vi "test_bench.vi"   [LabVIEW 2016]
types:
  T1 = cluster{"B":dbl[][], "Cline":dbl[][], "Kline":dbl[][], "Mline":dbl[][], "Alp0":dbl, "Alp1":dbl, "Gam0":dbl, "Gam1":dbl, "T_shift":dbl, "Numerator":dbl[], "Denominator":dbl[]}
  T2 = typedef "NI_LinSys_Model Typedefs.lvlib/CD State Space Model (MIMO).ctl" = cluster{"properties":T3, "A":dbl[][], "B":dbl[][], "C":dbl[][], "D":dbl[][], "StateNames":string[], "Transport Delay":dbl[][]}
  T3 = typedef "NI_LinSys_Model Typedefs.lvlib/CD General Elements.ctl" = cluster{"Model name":string, "Input names":string[], "Output names":string[], "Input Delays":dbl[], "Output Delays":dbl[], "Sampling Time":dbl, "Notes":string}
  T4 = typedef "NI_LinSys_Model Typedefs.lvlib/CD Transfer Function Model (MIMO).ctl" = cluster{"properties":T3, "transfer function(s)":T5[][]}
  T5 = typedef "NI_LinSys_Model Typedefs.lvlib/CD Transfer Function Model (SISO).ctl" = cluster{"Numerator":dbl[], "Denominator":dbl[], "delay":dbl}
  T6 = cluster{"SysD":T2, "sysDo":T2, "sysDi":T2, "sysDC":T4}
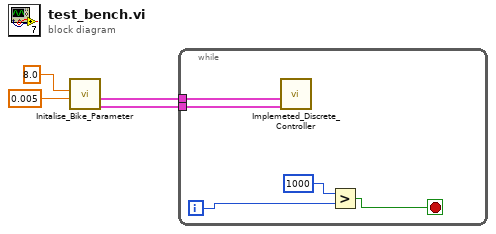
[diagram p0: block diagram]
diagram:
  n1 = call "Initalise_Bike_Parameter.vi"("Ts"=0.005, "Velocity"=8.0) -> ("Other variables"=w2:T1, "systems"=w3:T6)  [unwired: 7 in]
  n2 = while {
    tunnel: w3 -> [w8]
    tunnel: w2 -> [w9]
    i -> [w6]
    stop <- w7 stop-if-true
    n3 = call "Implemeted_Discrete_Controller.vi"("Other variables"=w9, "systems"=w8) -> ()  [unwired: 7 in, 3 out]
    n4 = Greater?(x=1000, y=w6) -> (0:w7:bool)
  }
